vi "PID Normalize Step Response.vi"(8 "start index":i32=10, 9 "length":i32=10, 11 "response signal":dbl[](array[numeric])) -> (0 "error code":i32, 1 "noise":dbl, 2 "step height":dbl, 3 "response norm":dbl[](array[numeric]), 4 "response offset":dbl)   [LabVIEW 2020, in "NI_PID_autopid.lvlib"]
uses:
  <vilib>/addons/control/pid/NI_PID_autopid.lvlib
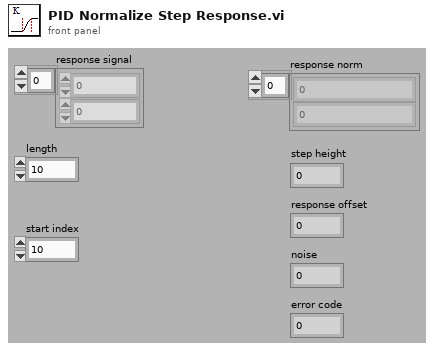
[diagram p1: front panel]
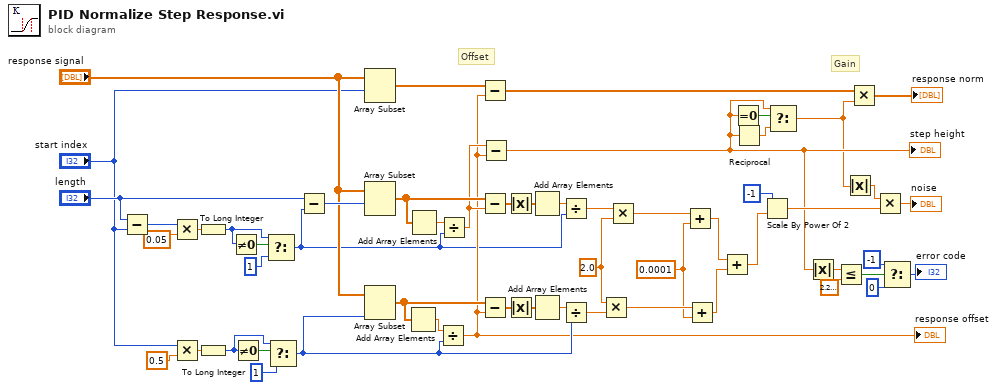
[diagram p0: block diagram]
diagram:
  w5 = 2.0 ("x")
  w6 = 0.0001 ("x*y")
  # "Gain"
  # "Offset"
  n1 = Subtract(x="length", y="start index") -> (x-y=w55:i32)
  n2 = Multiply(x=w55, y=0.05) -> (x*y=w53:dbl)
  n3 = Multiply(x="start index", y=0.5 ("x")) -> (x*y=w45:dbl)
  n4 = To Long Integer(number=w53) -> (32bit integer=w17:i32)
  n5 = To Long Integer(number=w45) -> (32bit integer=w21:i32)
  n6 = Not Equal To 0?(x=w17) -> (x != 0?=w18:bool)
  n7 = Not Equal To 0?(x=w21) -> (x != 0?=w23:bool)
  n8 = Select(t=w17, s=w18, f=1) -> (s? t:f=w7:i32)
  n9 = Select(t=w21, s=w23, f=1) -> (s? t:f=w20:i32)
  n10 = Subtract(x="length", y=w7) -> (x-y=w51:i32)
  n11 = Array Subset(array="response signal", index="start index") -> (w49:dbl[])  [unwired: 1 in]
  n12 = Array Subset(array="response signal", index=w51) -> (w38:dbl[])  [unwired: 1 in]
  n13 = Array Subset(array="response signal", length=w20) -> (w44:dbl[])  [unwired: 1 in]
  n14 = Add Array Elements(numeric array=w44) -> (sum=w9:dbl)
  n15 = Add Array Elements(numeric array=w38) -> (sum=w25:dbl)
  n16 = Divide(x=w9, y=w20) -> (x/y=w8:dbl)
  "response offset" <- w8
  n17 = Divide(x=w25, y=w7) -> (x/y=w37:dbl)
  n18 = Subtract(x=w49, y=w8) -> (x-y=w15:dbl[])
  n19 = Subtract(x=w38, y=w37) -> (x-y=w26:dbl[])
  n20 = Subtract(x=w44, y=w8) -> (x-y=w10:dbl[])
  n21 = Subtract(x=w37, y=w8) -> (x-y=w3:dbl)
  "step height" <- w3
  n22 = Absolute Value(x=w26) -> (abs(x)=w27:dbl[])
  n23 = Absolute Value(x=w10) -> (abs(x)=w11:dbl[])
  n24 = Add Array Elements(numeric array=w27) -> (sum=w28:dbl)
  n25 = Add Array Elements(numeric array=w11) -> (sum=w12:dbl)
  n26 = Divide(x=w28, y=w7) -> (x/y=w29:dbl)
  n27 = Divide(x=w12, y=w20) -> (x/y=w13:dbl)
  n28 = Multiply(x=w5, y=w13) -> (x*y=w14:dbl)
  n29 = Multiply(x=w29, y=w5) -> (x*y=w30:dbl)
  n30 = Add(x=w30, y=w6) -> (x+y=w33:dbl)
  n31 = Add(x=w14, y=w6) -> (x+y=w35:dbl)
  n32 = Add(x=w33, y=w35) -> (x+y=w36:dbl)
  n33 = Equal To 0?(x=w3) -> (x = 0?=w4:bool)
  n34 = Reciprocal(x=w3) -> (1/x=w2:dbl)
  n35 = Scale By Power Of 2(n=-1, x=w36) -> (x*2^n=w34:dbl)
  n36 = Select(t=w3, s=w4, f=w2) -> (s? t:f=w1:dbl)
  n37 = Absolute Value(x=w3) -> (abs(x)=w42:dbl)
  n38 = Less Or Equal?(x=w42, y=2.220446049250313e-16) -> (x <= y?=w40:bool)
  n39 = Absolute Value(x=w1) -> (abs(x)=w39:dbl)
  n40 = Multiply(x=w15, y=w1) -> (x*y=→"response norm":dbl[])
  n41 = Multiply(x=w39, y=w34) -> (x*y=→"noise":dbl)
  n42 = Select(t=-1, s=w40, f=0) -> (s? t:f=→"error code":i32)
